vi "Color Process Image.vi"(6 "Color Filter Array Phase":i32(ring) items=["BayerRed", "BayerBlue", "BayerGreenLeftOfRed", "BayerGreenLeftOfBlue"], 8 "error in (no error)":errorcluster, 9 "ImageData":refnum<k24>, 10 "Image Type":T1, 11 "Color Processor References":T2) -> (0 "error out":errorcluster, 2 "Color Data":u16[][][](array[numeric]))   [LabVIEW 2019]
uses:
  Color/Color Processor References.ctl
  Thor_Controls/Color Modes.ctl
  C:/code/ScientificCameraInterfaces/Installer/Scientific Camera Interfaces/LabVIEW/64_bit/Library_X64/Thorlabs.TSI.ImageDataInterfaces.dll
  code/ScientificCameraInterfaces/Installer/Scientific Camera Interfaces/LabVIEW/64_bit/Library_X64/Thorlabs.TSI.ImageDataInterfaces.dll
  C:/code/ScientificCameraInterfaces/Installer/Scientific Camera Interfaces/LabVIEW/64_bit/Library_X64/Thorlabs.TSI.ColorInterfaces.dll
  code/ScientificCameraInterfaces/Installer/Scientific Camera Interfaces/LabVIEW/64_bit/Library_X64/Thorlabs.TSI.ColorInterfaces.dll
  C:/code/ScientificCameraInterfaces/Installer/Scientific Camera Interfaces/LabVIEW/64_bit/Library_X64/Thorlabs.TSI.ColorProcessor.dll
  code/ScientificCameraInterfaces/Installer/Scientific Camera Interfaces/LabVIEW/64_bit/Library_X64/Thorlabs.TSI.ColorProcessor.dll
  C:/code/ScientificCameraInterfaces/Installer/Scientific Camera Interfaces/LabVIEW/64_bit/Library_X64/Thorlabs.TSI.Demosaicker.dll
  code/ScientificCameraInterfaces/Installer/Scientific Camera Interfaces/LabVIEW/64_bit/Library_X64/Thorlabs.TSI.Demosaicker.dll
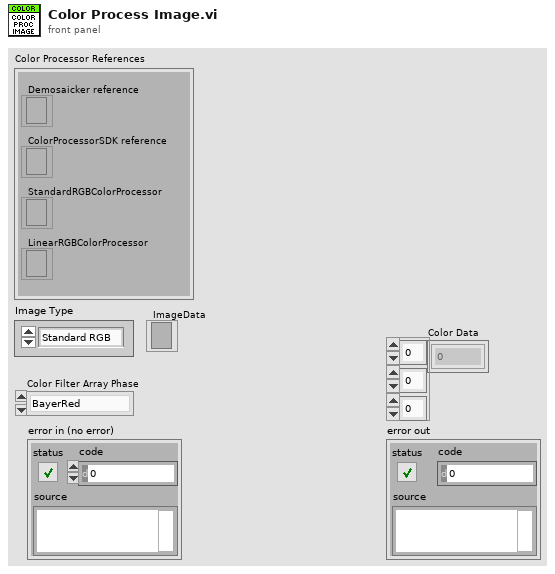
[diagram p1: front panel]
types:
  T1 = typedef "Color Modes.ctl" = enum16{"Standard RGB", "Linear RGB", "Unprocessed"}
  T2 = typedef "Color Processor References.ctl" = cluster{"Demosaicker reference":refnum<k24>, "ColorProcessorSDK reference":refnum<k24>, "StandardRGBColorProcessor":refnum<k24>, "LinearRGBColorProcessor":refnum<k24>}
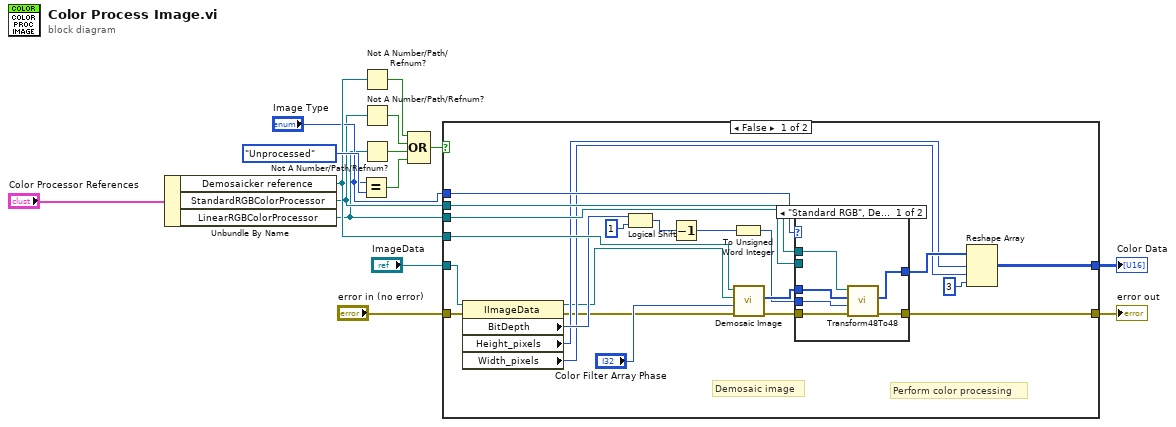
[diagram p0: block diagram]
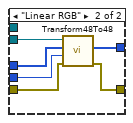
[diagram p2: hidden frame]
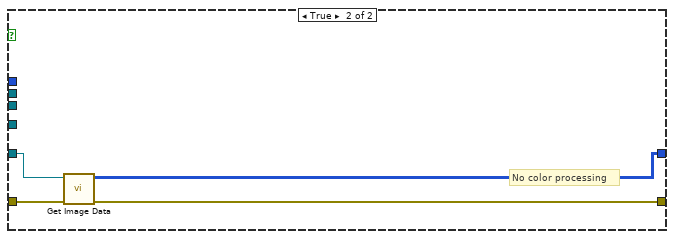
[diagram p3: hidden frame]
diagram:
  n1 = Unbundle By Name("Color Processor References") -> ("Demosaicker reference"=w6:refnum<k24>, "StandardRGBColorProcessor"=w4:refnum<k24>, "LinearRGBColorProcessor"=w3:refnum<k24>)
  n2 = Equal?(x="Image Type", y=Color_Modes."Unprocessed") -> (x = y?=w9:bool)
  n3 = Not A Number/Path/Refnum?(number/path/refnum=w6) -> (NaN/Path/Refnum?=w13:bool)
  n4 = Not A Number/Path/Refnum?(number/path/refnum=w4) -> (NaN/Path/Refnum?=w7:bool)
  n5 = Not A Number/Path/Refnum?(number/path/refnum=w3) -> (NaN/Path/Refnum?=w8:bool)
  n6 = Compound Arithmetic op=OR(w13, w7, w8, w9) -> (w12:bool)
  n7 = case shown="False" w12 {
    tunnel: "ImageData" -> [w30 w53]
    tunnel: "error in (no error)" -> [w18 w52]
    tunnel: [w20 w51] -> w2
    tunnel: w6 -> [w37 _]
    tunnel: "Image Type" -> [w35 _]
    tunnel: w4 -> [w34 _]
    tunnel: w3 -> [w33 _]
    tunnel: [w19 w50] -> w1
    frame False {
      # "Demosaic image"
      # "Perform color processing"
      n8 = property class="IImageData"(reference=w30, error in=w18) -> (reference out=w16:refnum<k24>, error out=w17:errorcluster, "BitDepth"=w28:i32, "Height_pixels"=w22:i32, "Width_pixels"=w21:i32)
      n9 = Logical Shift(y=w28, x=u32 1) -> (x << y=w27:u32)
      n10 = Decrement(x=w27) -> (x-1=w26:u32)
      n11 = To Unsigned Word Integer(number=w26) -> (unsigned 16bit integer=w25:u16)
      n12 = call "Demosaic Image.vi"("error in (no error)"=w17, "Color Filter Array Phase"="Color Filter Array Phase", "ImageData"=w16, "Demosaicker reference in"=w37) -> ("error out"=w32:errorcluster, "Demosaicked Data"=w31:u16[])  [unwired: 5 in, 1 out]
      n13 = case shown="\"Standard RGB\", Default" w35 {
        tunnel: w34 -> [w43 _]
        tunnel: w33 -> [_ w49]
        tunnel: w32 -> [w40 w48]
        tunnel: w31 -> [w42 w46]
        tunnel: w25 -> [w41 w47]
        tunnel: [w39 w44] -> w24
        tunnel: [w38 w45] -> w19
        frame "Standard RGB", Default {
          n14 = call "Transform48To48.vi"("error in (no error)"=w40, "Max Output Value"=w41, "Demosaicked Data"=w42, "ColorProcessor reference in"=w43) -> ("error out"=w38:errorcluster, "outputData"=w39:u16[])  [unwired: 5 in, 1 out]
        }
        frame "Linear RGB" {
          n15 = call "Transform48To48.vi"("error in (no error)"=w48, "Max Output Value"=w47, "Demosaicked Data"=w46, "ColorProcessor reference in"=w49) -> ("error out"=w45:errorcluster, "outputData"=w44:u16[])  [unwired: 5 in, 1 out]
        }
      }
      n16 = Reshape Array(w24, w22, w21, 3 ("dimension size")) -> (w20:u16[][][])
    }
    frame True {
      # "No color processing"
      n17 = call "Get Image Data.vi"("error in (no error)"=w52, "ImageData"=w53) -> ("error out"=w50:errorcluster, "Frame Data"=w51:u16[][][])  [unwired: 6 in, 2 out]
    }
  }
  "Color Data" <- w2
  "error out" <- w1
